vi "RTS Save Routine.vi"(5 "Setup Info Station 8":string[][](array[string]), 7 "TDMS Data Save Input":T1, 8 "error in (no error)":errorcluster, 9 "Save Status 8":bool, 10 "Custom Saved Titles":string[][](array[string]), 11 "Station Number":u8) -> (0 "error out":errorcluster, 3 "CSV Data Save Output":T1)   [LabVIEW 2016]
uses:
  Type Definitions/RTS TDMS Filename Locations.ctl
  Type Definitions/RTS Save References.ctl
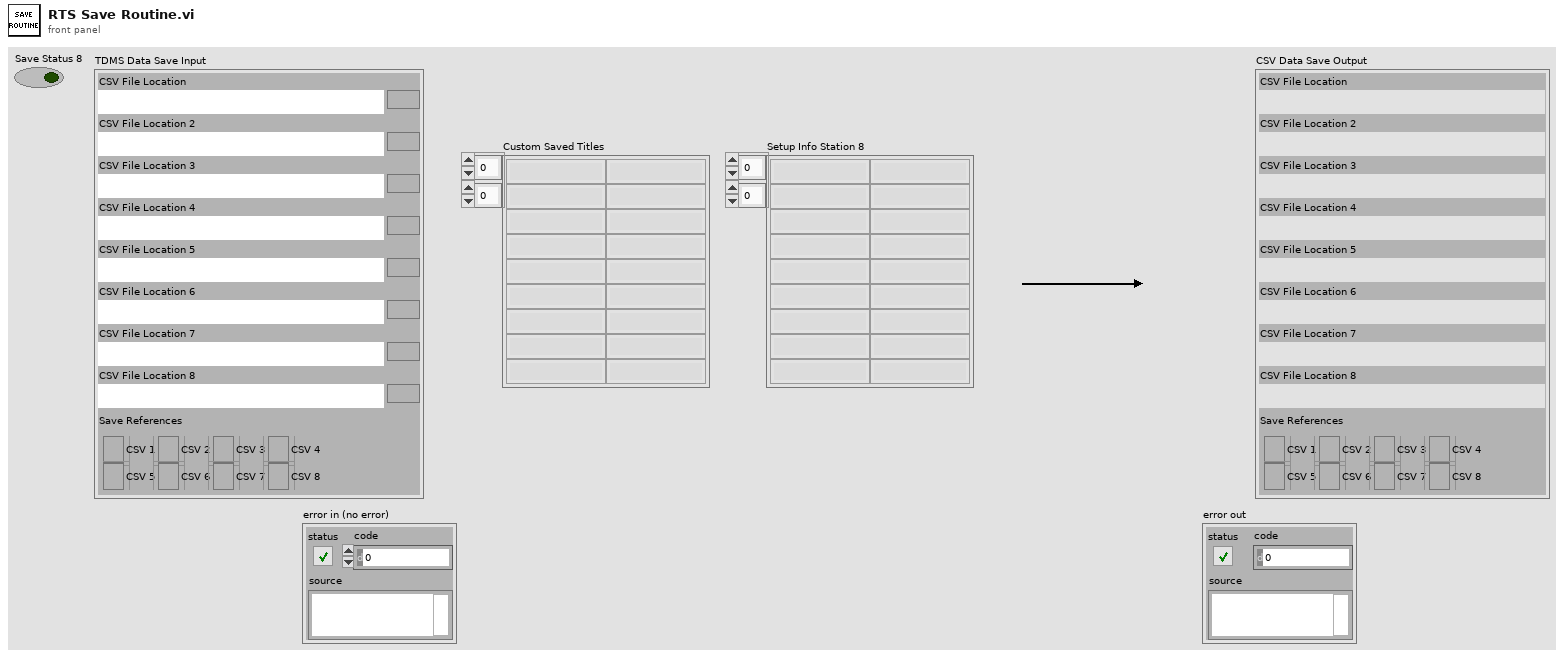
[diagram p1: front panel]
types:
  T1 = typedef "RTS TDMS Filename Locations.ctl" = cluster{"CSV File Location":path, "CSV File Location 2":path, "CSV File Location 3":path, "CSV File Location 4":path, "CSV File Location 5":path, "CSV File Location 6":path, "CSV File Location 7":path, "CSV File Location 8":path, "Save References":T2}
  T2 = typedef "RTS Save References.ctl" = cluster{"CSV 1":refnum<file>, "CSV 2":refnum<file>, "CSV 3":refnum<file>, "CSV 4":refnum<file>, "CSV 5":refnum<file>, "CSV 6":refnum<file>, "CSV 7":refnum<file>, "CSV 8":refnum<file>}
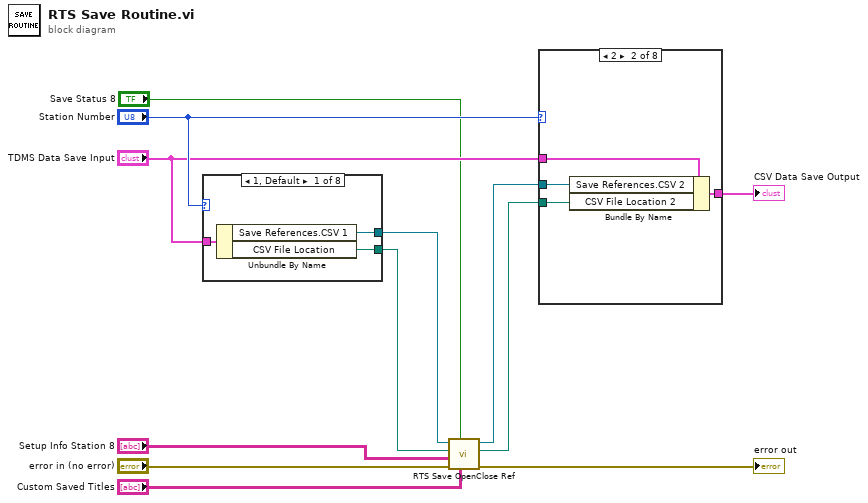
[diagram p0: block diagram]
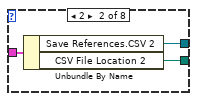
[diagram p2: hidden frame]
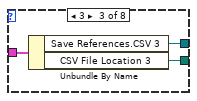
[diagram p3: hidden frame]
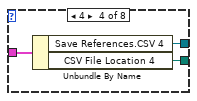
[diagram p4: hidden frame]
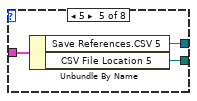
[diagram p5: hidden frame]
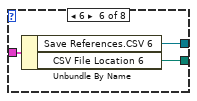
[diagram p6: hidden frame]
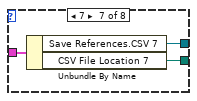
[diagram p7: hidden frame]
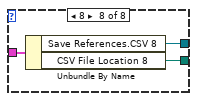
[diagram p8: hidden frame]
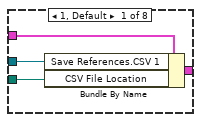
[diagram p9: hidden frame]
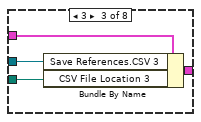
[diagram p10: hidden frame]
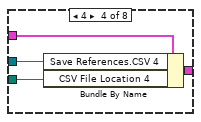
[diagram p11: hidden frame]
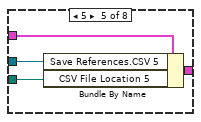
[diagram p12: hidden frame]
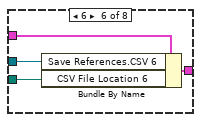
[diagram p13: hidden frame]
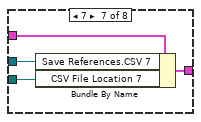
[diagram p14: hidden frame]
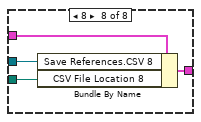
[diagram p15: hidden frame]
diagram:
  n1 = case shown="1, Default" "Station Number" {
    tunnel: "TDMS Data Save Input" -> [w15 w18 w21 w24 w27 w30 w33 w36]
    tunnel: [w14 w17 w20 w23 w26 w29 w32 w35] -> w12
    tunnel: [w13 w16 w19 w22 w25 w28 w31 w34] -> w11
    frame 1, Default {
      n2 = Unbundle By Name(w15) -> ("Save References.CSV 1"=w13:refnum<file>, "CSV File Location"=w14:path)
    }
    frame 2 {
      n3 = Unbundle By Name(w18) -> ("Save References.CSV 2"=w16:refnum<file>, "CSV File Location 2"=w17:path)
    }
    frame 3 {
      n4 = Unbundle By Name(w21) -> ("Save References.CSV 3"=w19:refnum<file>, "CSV File Location 3"=w20:path)
    }
    frame 4 {
      n5 = Unbundle By Name(w24) -> ("Save References.CSV 4"=w22:refnum<file>, "CSV File Location 4"=w23:path)
    }
    frame 5 {
      n6 = Unbundle By Name(w27) -> ("Save References.CSV 5"=w25:refnum<file>, "CSV File Location 5"=w26:path)
    }
    frame 6 {
      n7 = Unbundle By Name(w30) -> ("Save References.CSV 6"=w28:refnum<file>, "CSV File Location 6"=w29:path)
    }
    frame 7 {
      n8 = Unbundle By Name(w33) -> ("Save References.CSV 7"=w31:refnum<file>, "CSV File Location 7"=w32:path)
    }
    frame 8 {
      n9 = Unbundle By Name(w36) -> ("Save References.CSV 8"=w34:refnum<file>, "CSV File Location 8"=w35:path)
    }
  }
  n10 = call "RTS Save OpenClose Ref.vi"("Custom Saved Titles"="Custom Saved Titles", "Save Status 8"="Save Status 8", "error in (no error)"="error in (no error)", "Setup Info Station 8"="Setup Info Station 8", "CSV File Location 8"=w12, "Byte Stream File in"=w11) -> ("error out"=→"error out":errorcluster, "CSV File Location Output"=w7:path, "Byte Stream File out"=w6:refnum<file>)  [unwired: 3 in]
  n11 = case shown="2" "Station Number" {
    tunnel: "TDMS Data Save Input" -> [w40 w44 w48 w52 w56 w60 w64 w68]
    tunnel: [w39 w43 w47 w51 w55 w59 w63 w67] -> w3
    tunnel: w6 -> [w38 w42 w46 w50 w54 w58 w62 w66]
    tunnel: w7 -> [w37 w41 w45 w49 w53 w57 w61 w65]
    frame 1, Default {
      n12 = Bundle By Name(cluster=w40, "Save References.CSV 1"=w38, "CSV File Location"=w37) -> (w39:T1)
    }
    frame 2 {
      n13 = Bundle By Name(cluster=w44, "Save References.CSV 2"=w42, "CSV File Location 2"=w41) -> (w43:T1)
    }
    frame 3 {
      n14 = Bundle By Name(cluster=w48, "Save References.CSV 3"=w46, "CSV File Location 3"=w45) -> (w47:T1)
    }
    frame 4 {
      n15 = Bundle By Name(cluster=w52, "Save References.CSV 4"=w50, "CSV File Location 4"=w49) -> (w51:T1)
    }
    frame 5 {
      n16 = Bundle By Name(cluster=w56, "Save References.CSV 5"=w54, "CSV File Location 5"=w53) -> (w55:T1)
    }
    frame 6 {
      n17 = Bundle By Name(cluster=w60, "Save References.CSV 6"=w58, "CSV File Location 6"=w57) -> (w59:T1)
    }
    frame 7 {
      n18 = Bundle By Name(cluster=w64, "Save References.CSV 7"=w62, "CSV File Location 7"=w61) -> (w63:T1)
    }
    frame 8 {
      n19 = Bundle By Name(cluster=w68, "Save References.CSV 8"=w66, "CSV File Location 8"=w65) -> (w67:T1)
    }
  }
  "CSV Data Save Output" <- w3
